vi "Output Enable Write.vi"   [LabVIEW 2023, in "Power Supply.lvclass"]
uses:
  Power Supply.lvclass
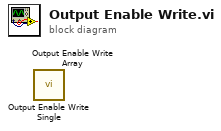
[diagram p0: block diagram]
diagram:
  n1 = call "Output Enable Write Single.vi"() -> ()  [unwired: 10 in, 2 out]
  n2 = call "Output Enable Write Array.vi"() -> ()  [unwired: 10 in, 2 out]
